vi "Audio File Tags Example.vi"() -> ()   [LabVIEW 2020]
doc: "Demonstrates reading tag data and embedded artwork from an audio file using G-Audio."
uses:
  Controls/Audio File Image.ctl
  Controls/Audio File Image Type.ctl
  <vilib>/picture/picture.llb/imagedata.ctl
  Controls/Text Encoding.ctl
  39f23256-a1b8-4f94-abd0-7b94a94a87d6.vi
  Audio Files/Polymorphic VIs/Get Audio File Tags (Path).vi
  G-Audio.lvlib
panel:
  in  "File Path":path
  in  "Embedded Artwork":u16(ring) items=["Cover (front)", "Media (e.g. label side of CD)"]
  out "Tags":T1
  in  "Stop":bool
  out "Picture":picture
  out "Raw Tags":cluster{"Field":string, "Value":string}[](array[cluster])
  out "Reflection":picture
  # "Instructions:\n1. Run the VI.\n2. Select an audio file to read the tag data from.\n3. Use the Embedded Artwork ring to select which artwork to view (if any).\n4. Use File Path to select another audio file to read tag data from."
  # "Embedded images can be jpg, png, bmp, or gif format. Images with transparency are loaded as 32-bit RGBA. A one 1-bit mask is then calculated, as LabVIEW images don't support a true alpha channel."
  # "NOTE: Value indicators have been forced to display unicode text, and require strings with UTF-16 LE encoding. The Audio File Read Tags.vi function is configured to return UTF-16 LE encoded values. Be warned that LabVIEW's unicode string support is lacking, and should be used for display only."
  # "G"
  # "-Audio"
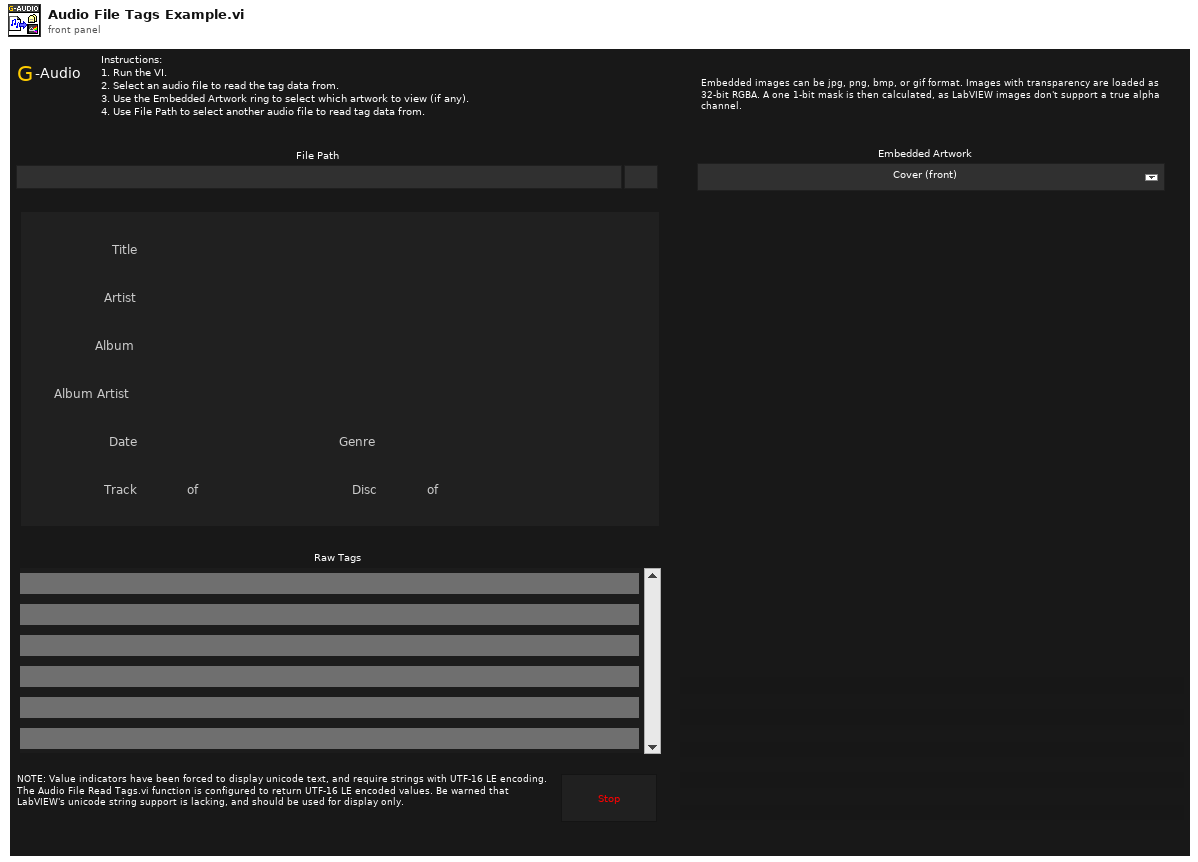
[diagram p1: front panel]
types:
  T1 = cluster{"Artist":string, "Album":string, "Title":string, "Album Artist":string, "Track":string, "Disc":string, "Genre":string, "Date":string, "Track Total":string, "Disc Total":string}
  T2 = typedef "G-Audio.lvlib/Audio File Image.ctl" = cluster{"Type":T3, "Pixmap":T4}
  T3 = typedef "G-Audio.lvlib/Audio File Image Type.ctl" = enum32{"Other", "32x32 pixels 'file icon' (PNG only)", "Other file icon", "Cover (front)", "Cover (back)", "Leaflet page", "Media (e.g. label side of CD)", "Lead artist/lead performer/soloist", "Artist/performer", "Conductor", "Band/Orchestra", "Composer", "Lyricist/text writer", "Recording Location", "During recording", "During performance", "Movie/video screen capture", "A bright coloured fish", "Illustration", "Band/artist logotype", "Publisher/Studio logotype"}
  T4 = typedef "imagedata.ctl" = cluster{"image type":i32, "image depth":i32, "image":u8[], "mask":u8[], "colors":u32[], "Rectangle":cluster{"left":i16, "top":i16, "right":i16, "bottom":i16}}
  T5 = typedef "G-Audio.lvlib/Text Encoding.ctl" = enum16{"ASCII", "UTF-8", "UTF-16 LE"}
  T6 = typedef "G-Audio.lvlib/Audio File Tag.ctl" = cluster{"Field":string, "Value":string}
  T7 = typedef "LVBoundsTypeDef.ctl" = cluster{"Width":u32, "Height":u32}
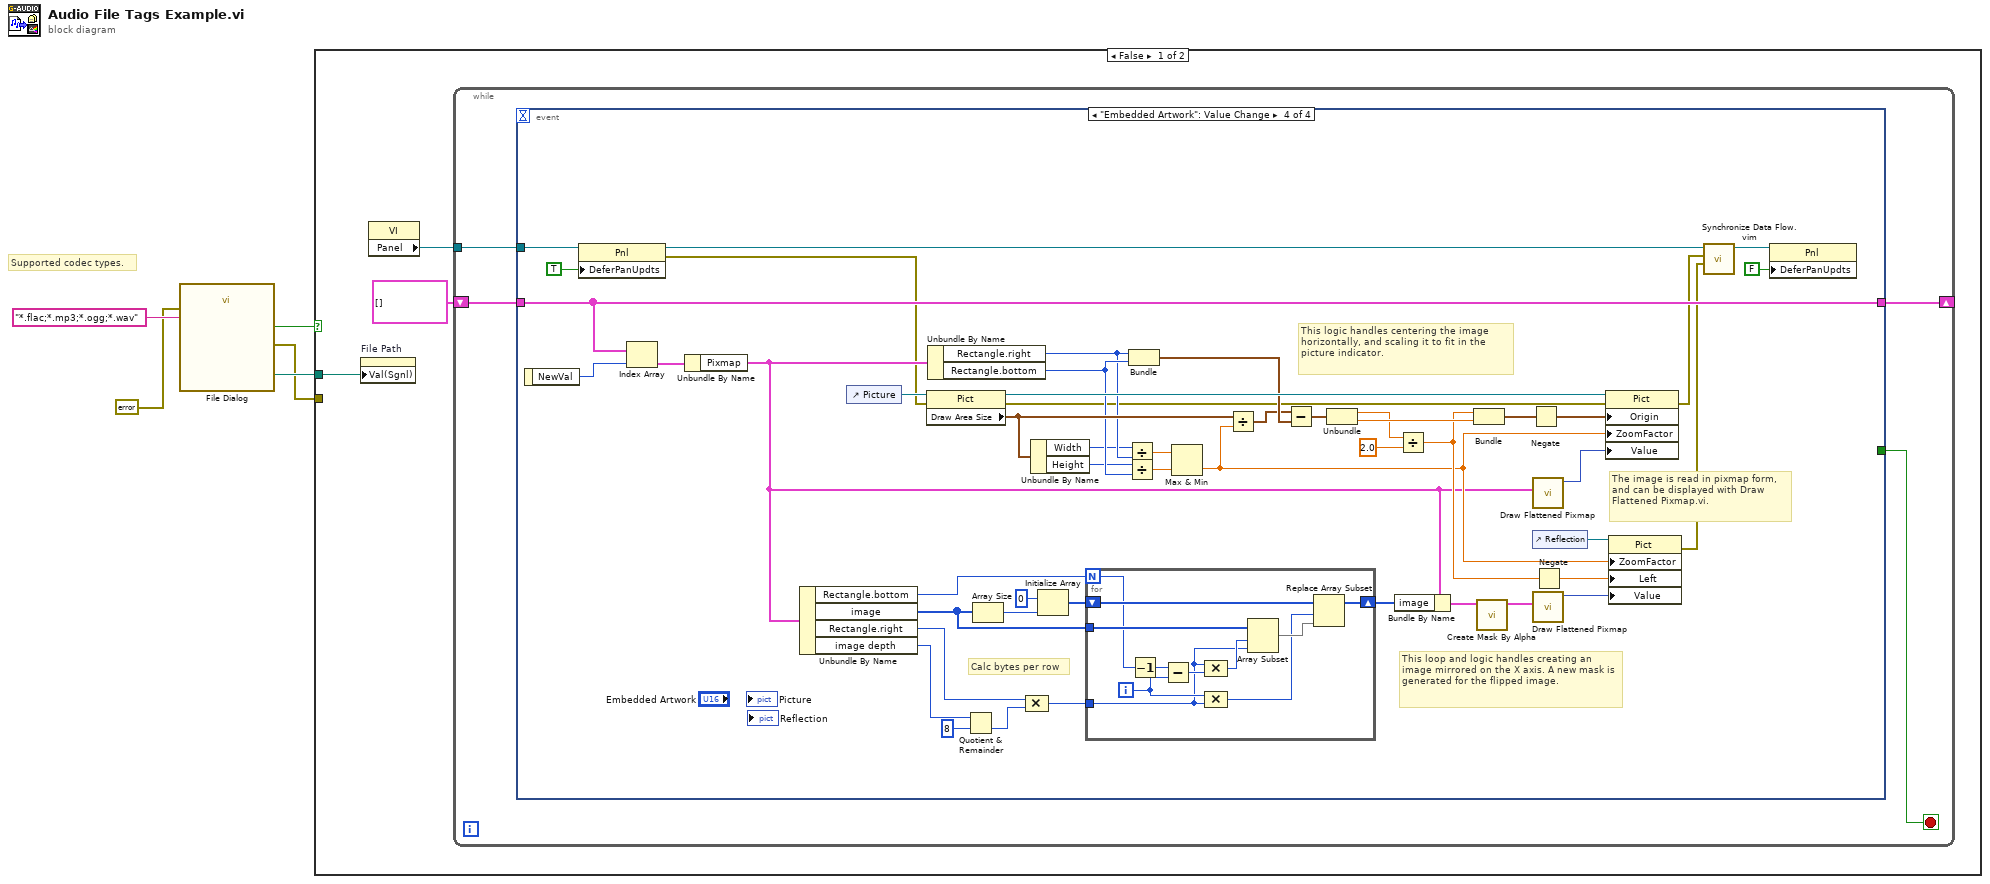
[diagram p0: block diagram]
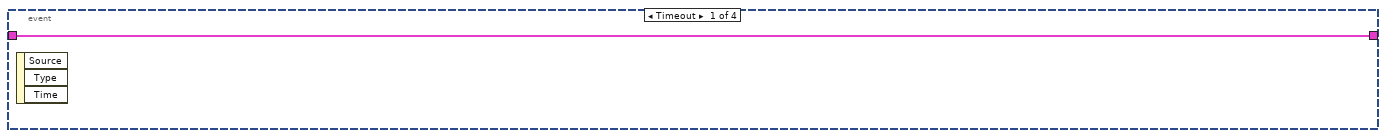
[diagram p2: hidden frame]
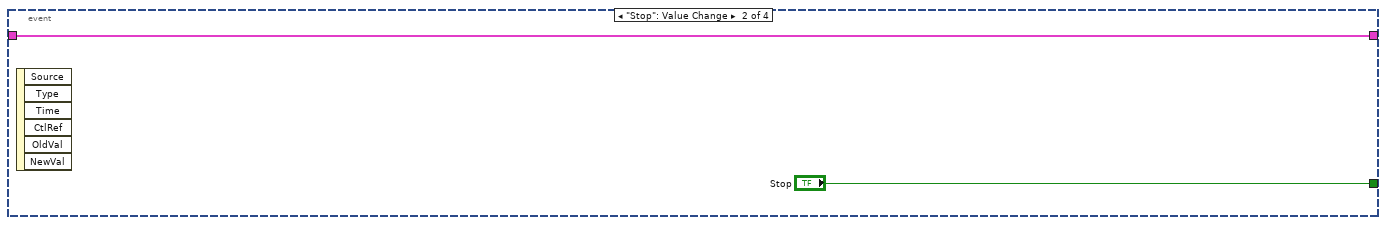
[diagram p3: hidden frame]
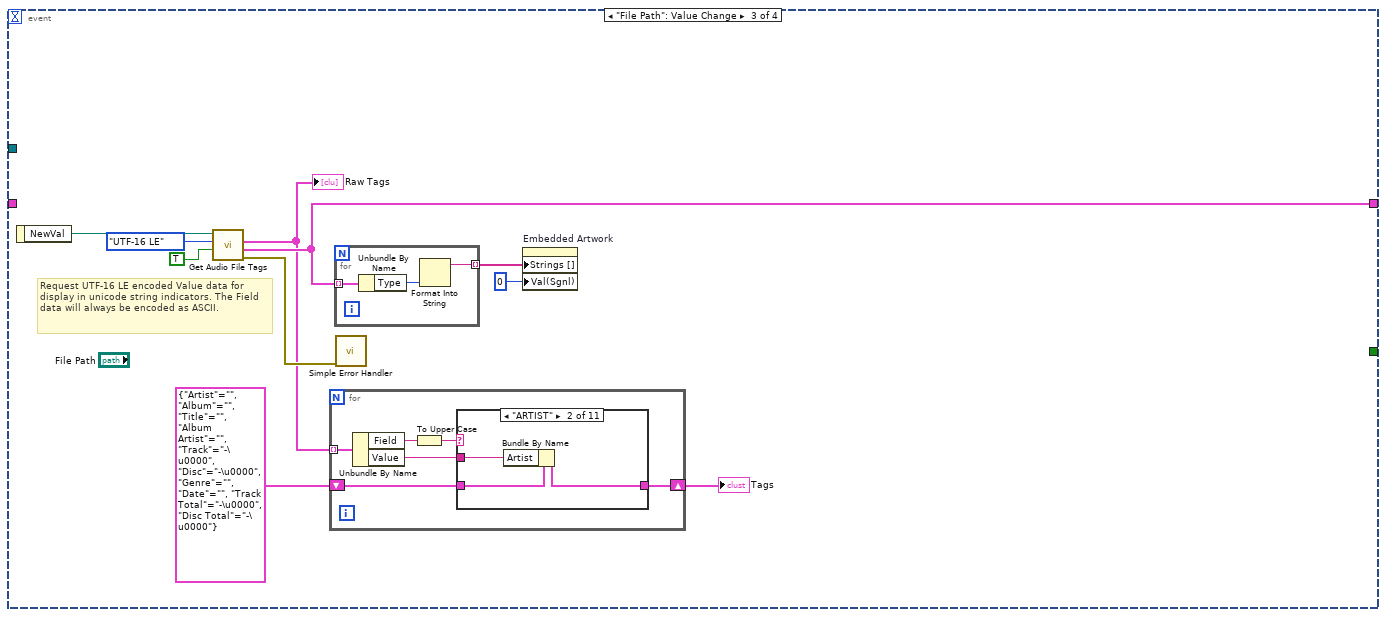
[diagram p4: hidden frame]
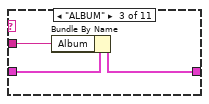
[diagram p6: hidden frame]
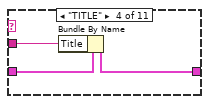
[diagram p7: hidden frame]
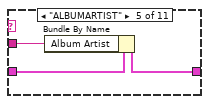
[diagram p8: hidden frame]
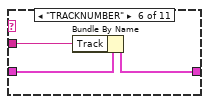
[diagram p9: hidden frame]
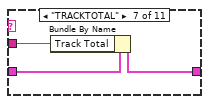
[diagram p10: hidden frame]
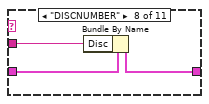
[diagram p11: hidden frame]
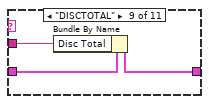
[diagram p12: hidden frame]
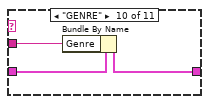
[diagram p13: hidden frame]
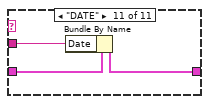
[diagram p14: hidden frame]
diagram:
  # "Supported codec types."
  n1 = call "File Dialog"("error in"=errorcluster {"status"=FALSE, "code"=0, "source"=""} ("error out"), "pattern (all files)"="*.flac;*.mp3;*.ogg;*.wav") -> ("selected path"=w4:path, "cancelled"=w3:bool, "error out"=w2:errorcluster)  [unwired: 10 in, 1 out]
  n2 = case shown="False" w3 {
    tunnel: w4 -> [w7 _]
    tunnel: w2 -> [_ _]
    frame False {
      n3 = property on="File Path" class="Path"("Val(Sgnl)"=w7) -> ()  [unwired: 2 in, 2 out]
      n4 = property class="VI"() -> ("Panel"=w6:refnum<vi>)  [unwired: 2 in, 2 out]
      n5 = while {
        shift-right: [w11] -> _
        shift-left: T2[] [] ("Pictures") -> [w10]
        tunnel: w6 -> [w9]
        stop <- w12 stop-if-true
        n6 = event shown="[3] \"Embedded Artwork\": Value Change" {
          selector: _ -> [_ _ _ _]
          dyn-events: _ -> [_ _ _ _]
          timeout: _ -> [_ _ _ _]
          tunnel: [_ "Stop" _ _] -> w12
          tunnel: [w13 w14 w23 w99] -> w11
          tunnel: w10 -> [w13 w14 _ w99]
          tunnel: w9 -> [_ _ _ w76]
          event Timeout {
            n7 = event-data() -> ()  [unwired: 1 in, 3 out]
          }
          event "Stop": Value Change {
            n8 = event-data() -> ()  [unwired: 1 in, 6 out]
          }
          event "File Path": Value Change {
            # "Request UTF-16 LE encoded Value data for display in unicode string indicators. The Field data will always be encoded as ASCII."
            n9 = event-data() -> ("NewVal"=w22:path)  [unwired: 1 in]
            n10 = call-poly "Get Audio File Tags.vi"("Read Pictures? (F)"=TRUE, "Encoding (ASCII)"=Text_Encoding."UTF-16 LE", "Path In"=w22) -> ("error out"=w21:errorcluster, "Pictures"=w23:T2[], "Tags"=w16:T6[])  [unwired: 5 in, 1 out]
            "Raw Tags" <- w16
            n11 = for {
              tunnel: w16 -> [w31] mode=indexing
              shift-right: [w26] -> w19
              shift-left: T1 {"Artist"="", "Album"="", "Title"="", "Album Artist"="", "Track"="-\u0000", "Disc"="-\u0000", "Genre"="", "Date"="", "Track Total"="-\u0000", "Disc Total"="-\u0000"} ("Tags") -> [w27]
              n12 = Unbundle By Name(w31) -> ("Field"=w30:string, "Value"=w29:string)
              n13 = To Upper Case(1:w30) -> (0:w28:string)
              n14 = case shown="\"ARTIST\"" w28 {
                tunnel: w29 -> [_ w33 w36 w39 w42 w45 w48 w51 w54 w57 w60]
                tunnel: w27 -> [w32 w35 w38 w41 w44 w46 w49 w52 w55 w59 w62]
                tunnel: [w32 w34 w37 w40 w43 w47 w50 w53 w56 w58 w61] -> w26
                frame Default {
                }
                frame "ARTIST" {
                  n15 = Bundle By Name(cluster=w35, "Artist"=w33) -> (w34:T1)
                }
                frame "ALBUM" {
                  n16 = Bundle By Name(cluster=w38, "Album"=w36) -> (w37:T1)
                }
                frame "TITLE" {
                  n17 = Bundle By Name(cluster=w41, "Title"=w39) -> (w40:T1)
                }
                frame "ALBUMARTIST" {
                  n18 = Bundle By Name(cluster=w44, "Album Artist"=w42) -> (w43:T1)
                }
                frame "TRACKNUMBER" {
                  n19 = Bundle By Name(cluster=w46, "Track"=w45) -> (w47:T1)
                }
                frame "TRACKTOTAL" {
                  n20 = Bundle By Name(cluster=w49, "Track Total"=w48) -> (w50:T1)
                }
                frame "DISCNUMBER" {
                  n21 = Bundle By Name(cluster=w52, "Disc"=w51) -> (w53:T1)
                }
                frame "DISCTOTAL" {
                  n22 = Bundle By Name(cluster=w55, "Disc Total"=w54) -> (w56:T1)
                }
                frame "GENRE" {
                  n23 = Bundle By Name(cluster=w59, "Genre"=w57) -> (w58:T1)
                }
                frame "DATE" {
                  n24 = Bundle By Name(cluster=w62, "Date"=w60) -> (w61:T1)
                }
              }
            }
            "Tags" <- w19
            n25 = for {
              tunnel: w23 -> [w65] mode=indexing
              tunnel: [w63] -> w18 mode=indexing
              n26 = Unbundle By Name(w65) -> ("Type"=w64:T3)
              n27 = Format Into String(w64) -> (resulting string=w63:string)  [unwired: 3 in, 1 out]
            }
            n28 = call <vilib>:"Simple Error Handler.vi"("error in (no error)"=w21) -> ()  [unwired: 4 in, 5 out]
            n29 = property on="Embedded Artwork" class="Ring (strict)"("Strings []"=w18, "Val(Sgnl)"=u16 0 ("Value (Signaling)")) -> ()  [unwired: 2 in, 2 out]
          }
          event "Embedded Artwork": Value Change {
            # "Calc bytes per row"
            # "This loop and logic handles creating an image mirrored on the X axis. A new mask is generated for the flipped image."
            # "This logic handles centering the image horizontally, and scaling it to fit in the picture indicator."
            # "The image is read in pixmap form, and can be displayed with Draw Flattened Pixmap.vi."
            n30 = event-data() -> ("NewVal"=w100:u16)  [unwired: 1 in]
            n31 = property class="Pnl"(reference=w76, "DeferPanUpdts"=TRUE ("Defer Panel Updates")) -> (reference out=w68:refnum<vi>, error out=w66:errorcluster)  [unwired: 1 in]
            n32 = Index Array(array=w99, index=w100) -> (element=w101:T2)
            n33 = Unbundle By Name(w101) -> ("Pixmap"=w73:T4)
            n34 = Unbundle By Name(w73) -> ("Rectangle.bottom"=w90:i16, "image"=w88:u8[], "Rectangle.right"=w81:i16, "image depth"=w80:i32)
            n35 = control-ref of="Picture"() -> (w102:refnum<vi>)
            n36 = property on="Property Node" class="Pict"(reference=w102, error in=w66) -> (reference out=w114:refnum<vi>, error out=w107:errorcluster, "Draw Area Size"=w113:T7)
            n37 = Unbundle By Name(w73) -> ("Rectangle.right"=w109:i16, "Rectangle.bottom"=w110:i16)
            n38 = Quotient & Remainder(x=w80, y=8) -> (floor(x/y)=w78:i32)  [unwired: 1 out]
            n39 = Array Size(array=w88) -> (size(s)=w92:i32)
            n40 = Compound Arithmetic op=MULTIPLY(w81, w78) -> (w77:i32)
            n41 = Unbundle By Name(w113) -> ("Width"=w103:u32, "Height"=w104:u32)
            n42 = Initialize Array(u8 0, w92) -> (w89:u8[])
            n43 = for {
              N: w90 -> [w121]
              shift-right: [w123] -> w87
              shift-left: w89 -> [w124]
              tunnel: w88 -> [w125]
              tunnel: w77 -> [w115]
              i -> [w120]
              n44 = Decrement(x=w121) -> (x-1=w119:i32)
              n45 = Subtract(x=w119, y=w120) -> (x-y=w118:i32)
              n46 = Compound Arithmetic op=MULTIPLY(w115, w118) -> (w116:i32)
              n47 = Compound Arithmetic op=MULTIPLY(w120, w115) -> (w117:i32)
              n48 = Array Subset(array=w125, index=w116, length=w115) -> (w122:u8[])
              n49 = Replace Array Subset(array=w124, new element=w122, index=w117) -> (w123:u8[])
            }
            n50 = Divide(x=w103, y=w109) -> (x/y=w105:dbl)
            n51 = Divide(x=w104, y=w110) -> (x/y=w106:dbl)
            n52 = Bundle("right"=w109, "bottom"=w110) -> (w111:cluster{"right":i16, "bottom":i16})  [unwired: 1 in]
            n53 = Max & Min(x=w105, y=w106) -> (min(x,y)=w74:dbl)  [unwired: 1 out]
            n54 = Divide(x=w113, y=w74) -> (x/y=w108:cluster{"Width":dbl, "Height":dbl})
            n55 = Subtract(x=w108, y=w111) -> (x-y=w98:cluster{dbl, dbl})
            n56 = Unbundle(w98) -> (w95:dbl, w97:dbl)
            n57 = Bundle By Name(cluster=w73, "image"=w87) -> (w83:T4)
            n58 = Divide(x=w95, y=2.0) -> (x/y=w85:dbl)
            n59 = Bundle(w85, w97) -> (w96:cluster{dbl, dbl})  [unwired: 1 in]
            n60 = call <vilib>:"Create Mask By Alpha.vi"("image data"=w83) -> ("masked image data"=w82:T4)  [unwired: 10 in]
            n61 = Negate(x=w96) -> (-x=w112:cluster{dbl, dbl})
            n62 = call <vilib>:"Draw Flattened Pixmap.vi"("image data"=w73) -> ("new picture"=w72:picture)  [unwired: 8 in]
            n63 = control-ref of="Reflection"() -> (w93:refnum<vi>)
            n64 = call <vilib>:"Draw Flattened Pixmap.vi"("image data"=w82) -> ("new picture"=w86:picture)  [unwired: 8 in]
            n65 = Negate(x=w85) -> (-x=w84:dbl)
            n66 = property on="Property Node" class="Pict"(reference=w114, error in=w107, "Origin"=w112, "ZoomFactor"=w74, "Value"=w72) -> (error out=w70:errorcluster)  [unwired: 1 out]
            n67 = property on="Property Node" class="Pict"(reference=w93, "ZoomFactor"=w74, "Left"=w84, "Value"=w86) -> (error out=w69:errorcluster)  [unwired: 1 in, 1 out]
            n68 = call "Synchronize Data Flow.vim"("input 3"=w69, "input 2"=w70, "input 1"=w68) -> ("output 1"=w67:refnum<vi>)  [unwired: 1 in, 3 out]
            n69 = property class="Pnl"(reference=w67, "DeferPanUpdts"=FALSE ("Defer Panel Updates")) -> ()  [unwired: 1 in, 2 out]
          }
        }
      }
    }
    frame True {
    }
  }
